vi "Read Retardance.vi"(8 "errorIN":errorcluster caption="Error", 11 "LCD in":refnum<class "LCD Retarder.lvclass">) -> (0 "errorOUT":errorcluster caption="Error out", 2 "Retardance out":dbl, 3 "LCD out":refnum<class "LCD Retarder.lvclass">)   [LabVIEW 2015, in "LCD Retarder.lvclass"]
uses:
  LCD Retarder.lvclass
  LCD Retarder.lvclass/LCD Retarder.ctl
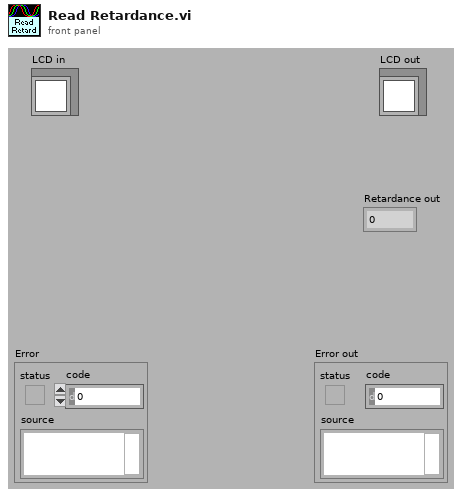
[diagram p1: front panel]
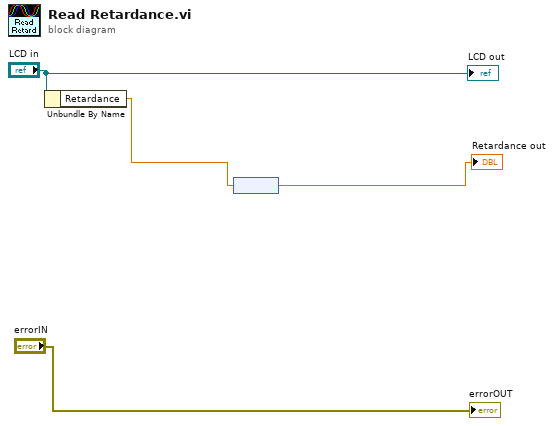
[diagram p0: block diagram]
diagram:
  n1 = Unbundle By Name("LCD in") -> ("Retardance"=w3:dbl[unit])
  n2 = node(w3) -> (→"Retardance out":dbl)
  "errorOUT" <- "errorIN"
  "LCD out" <- "LCD in"
